vi "Configure Output Parameters 2.vi"(0 "VISA resource name":refnum<visa-resource-name>, 1 "Unit Address (1)":u8=1, 5 "Enable Sensor Break (False:Safe)":bool, 7 "Safe Output Value (0)":sgl format="%.1g", 9 "The Output Power Sensor Break (0)":sgl format="%.1g", 11 "error in (no error)":errorcluster, 12 "Enable Forced Manual Output (False:Track)":bool, 13 "Feedforward Type (0:No)":u8(ring) items=["No", "Remote", "SP", "PV"]) -> (4 "VISA resource name out":refnum<visa-resource-name>, 15 "error out":errorcluster)   [LabVIEW 2014, in "Eurotherm 35xx Series.lvlib"]
doc: "This VI sets Output Parameters."
uses:
  <instrlib>/Eurotherm 35xx Series/Eurotherm 35xx Series.lvlib
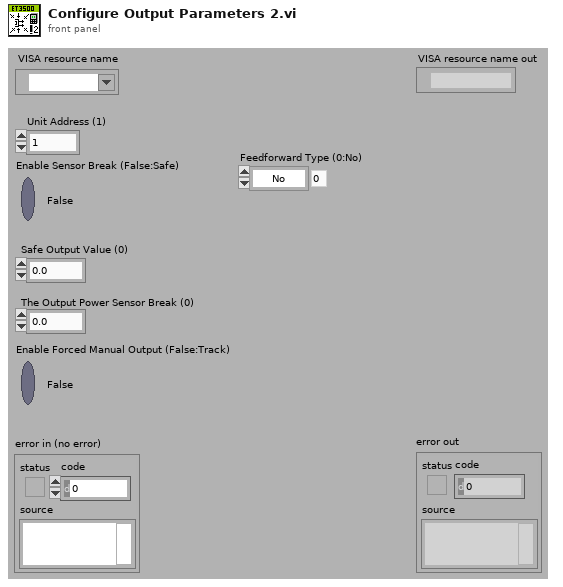
[diagram p1: front panel]
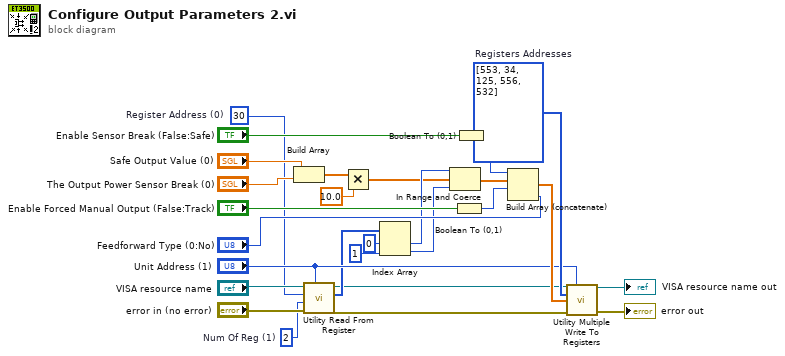
[diagram p0: block diagram]
diagram:
  w12 = u16 30  # Register Address (0)
  w13 = u16 2  # Num Of Reg (1)
  w20 = u16[] [553, 34, 125, 556, 532]  # Registers Addresses
  n1 = Build Array("Safe Output Value (0)", "The Output Power Sensor Break (0)") -> (w3:sgl[])
  n2 = call <instrlib>:"Utility Read From Register.vi"("Unit Address (1)"="Unit Address (1)", "error in (no error)"="error in (no error)", "Num Of Reg (1)"=w13, "Register Address (0)"=w12, "VISA resource name"="VISA resource name") -> ("error out"=w1:errorcluster, "Data"=w11:i16[], "VISA resource name out"=w2:refnum<visa-resource-name>)  [unwired: 4 in]
  n3 = Multiply(x=w3, y=sgl 10.0 ("Safe Output Value (0)")) -> (x*y=w6:sgl[])
  n4 = Index Array(array=w11, index #1=0 ("index"), index #2=1 ("index")) -> (element #1=w8:i16, element #2=w7:i16)
  n5 = In Range and Coerce(upper limit=w8, x=w6, lower limit=w7) -> (coerced(x)=w5:sgl[])  [unwired: 1 out]
  n6 = Boolean To (0,1)(Boolean="Enable Forced Manual Output (False:Track)") -> (0, 1=w23:i16)
  n7 = Boolean To (0,1)(Boolean="Enable Sensor Break (False:Safe)") -> (0, 1=w16:i16)
  n8 = Build Array (concatenate)(w16, w5, w23, "Feedforward Type (0:No)") -> (w21:sgl[])
  n9 = call <instrlib>:"Utility Multiple Write To Registers.vi"("VISA resource name"=w2, "Unit Address (1)"="Unit Address (1)", "Registers Addresses (0)"=w20, "Data (0)"=w21, "error in (no error)"=w1) -> ("VISA resource name out"=→"VISA resource name out":refnum<visa-resource-name>, "error out"=→"error out":errorcluster)  [unwired: 9 in]
